vi "数字量输入配置.vi"() -> ()   [LabVIEW 2010] (continued)
              n2465 = local write "单选_第17路"(w82) -> ()
              n2466 = local write "单选_第18路"(w82) -> ()
              n2467 = local write "单选_第19路"(w82) -> ()
              n2468 = local write "单选_第20路"(w82) -> ()
              n2469 = local write "单选_第21路"(w82) -> ()
              n2470 = local write "单选_第22路"(w82) -> ()
              n2471 = local write "单选_第23路"(w82) -> ()
              n2472 = local write "单选_第24路"(w82) -> ()
              n2473 = local write "单选_第25路"(w82) -> ()
              n2474 = local write "单选_第26路"(w83) -> ()
              n2475 = local write "单选_第27路"(w83) -> ()
              n2476 = local write "单选_第28路"(w83) -> ()
              n2477 = local write "单选_第29路"(w83) -> ()
              n2478 = local write "单选_第30路"(w83) -> ()
              n2479 = local write "单选_第31路"(w83) -> ()
              n2480 = local write "单选_第32路"(w83) -> ()
              n2481 = local write "单选_第33路"(w83) -> ()
              n2482 = local write "单选_第34路"(w83) -> ()
              n2483 = local write "单选_第35路"(w83) -> ()
              n2484 = local write "单选_第36路"(w83) -> ()
              n2485 = local write "单选_第37路"(w83) -> ()
              n2486 = local write "单选_第38路"(w83) -> ()
              n2487 = local write "单选_第39路"(w83) -> ()
              n2488 = local write "单选_第40路"(w83) -> ()
              n2489 = local write "单选_第41路"(w83) -> ()
              n2490 = local write "单选_第42路"(w83) -> ()
              n2491 = local write "单选_第43路"(w83) -> ()
              n2492 = local write "单选_第44路"(w83) -> ()
              n2493 = local write "单选_第45路"(w83) -> ()
              n2494 = local write "单选_第46路"(w83) -> ()
              n2495 = local write "单选_第47路"(w83) -> ()
              n2496 = local write "单选_第48路"(w83) -> ()
              n2497 = local write "单选_第49路"(w83) -> ()
              n2498 = local write "单选_第50路"(w83) -> ()
              n2499 = local write "单选_第51路"(w83) -> ()
              n2500 = local write "单选_第52路"(w83) -> ()
              n2501 = local write "单选_第53路"(w83) -> ()
              n2502 = local write "单选_第54路"(w83) -> ()
              n2503 = local write "单选_第55路"(w83) -> ()
              n2504 = local write "单选_第56路"(w83) -> ()
              n2505 = local write "单选_第57路"(w83) -> ()
              n2506 = local write "单选_第58路"(w83) -> ()
              n2507 = local write "单选_第59路"(w83) -> ()
              n2508 = local write "单选_第60路"(w83) -> ()
              n2509 = local write "单选_第61路"(w83) -> ()
              n2510 = local write "单选_第62路"(w83) -> ()
              n2511 = local write "单选_第63路"(w83) -> ()
              n2512 = local write "单选_第64路"(w83) -> ()
              n2513 = local write "单选_第71路"(w83) -> ()
              n2514 = local write "单选_第79路"(w83) -> ()
              n2515 = local write "单选_第65路"(w83) -> ()
              n2516 = local write "单选_第66路"(w83) -> ()
              n2517 = local write "单选_第67路"(w83) -> ()
              n2518 = local write "单选_第68路"(w83) -> ()
              n2519 = local write "单选_第69路"(w83) -> ()
              n2520 = local write "单选_第70路"(w83) -> ()
              n2521 = local write "单选_第72路"(w83) -> ()
              n2522 = local write "单选_第73路"(w83) -> ()
              n2523 = local write "单选_第74路"(w83) -> ()
              n2524 = local write "单选_第75路"(w83) -> ()
              n2525 = local write "单选_第76路"(w83) -> ()
              n2526 = local write "单选_第77路"(w83) -> ()
              n2527 = local write "单选_第78路"(w83) -> ()
              n2528 = local write "单选_第80路"(w83) -> ()
            }
            frame 26 {
              w84 = TRUE
              w85 = FALSE ("单选_第41路")
              n2529 = local write "单选_第1路"(w84) -> ()
              n2530 = local write "单选_第2路"(w84) -> ()
              n2531 = local write "单选_第3路"(w84) -> ()
              n2532 = local write "单选_第4路"(w84) -> ()
              n2533 = local write "单选_第5路"(w84) -> ()
              n2534 = local write "单选_第6路"(w84) -> ()
              n2535 = local write "单选_第7路"(w84) -> ()
              n2536 = local write "单选_第8路"(w84) -> ()
              n2537 = local write "单选_第9路"(w84) -> ()
              n2538 = local write "单选_第10路"(w84) -> ()
              n2539 = local write "单选_第11路"(w84) -> ()
              n2540 = local write "单选_第12路"(w84) -> ()
              n2541 = local write "单选_第13路"(w84) -> ()
              n2542 = local write "单选_第14路"(w84) -> ()
              n2543 = local write "单选_第15路"(w84) -> ()
              n2544 = local write "单选_第16路"(w84) -> ()
              n2545 = local write "单选_第17路"(w84) -> ()
              n2546 = local write "单选_第18路"(w84) -> ()
              n2547 = local write "单选_第19路"(w84) -> ()
              n2548 = local write "单选_第20路"(w84) -> ()
              n2549 = local write "单选_第21路"(w84) -> ()
              n2550 = local write "单选_第22路"(w84) -> ()
              n2551 = local write "单选_第23路"(w84) -> ()
              n2552 = local write "单选_第24路"(w84) -> ()
              n2553 = local write "单选_第25路"(w84) -> ()
              n2554 = local write "单选_第26路"(w84) -> ()
              n2555 = local write "单选_第27路"(w85) -> ()
              n2556 = local write "单选_第28路"(w85) -> ()
              n2557 = local write "单选_第29路"(w85) -> ()
              n2558 = local write "单选_第30路"(w85) -> ()
              n2559 = local write "单选_第31路"(w85) -> ()
              n2560 = local write "单选_第32路"(w85) -> ()
              n2561 = local write "单选_第33路"(w85) -> ()
              n2562 = local write "单选_第34路"(w85) -> ()
              n2563 = local write "单选_第35路"(w85) -> ()
              n2564 = local write "单选_第36路"(w85) -> ()
              n2565 = local write "单选_第37路"(w85) -> ()
              n2566 = local write "单选_第38路"(w85) -> ()
              n2567 = local write "单选_第39路"(w85) -> ()
              n2568 = local write "单选_第40路"(w85) -> ()
              n2569 = local write "单选_第41路"(w85) -> ()
              n2570 = local write "单选_第42路"(w85) -> ()
              n2571 = local write "单选_第43路"(w85) -> ()
              n2572 = local write "单选_第44路"(w85) -> ()
              n2573 = local write "单选_第45路"(w85) -> ()
              n2574 = local write "单选_第46路"(w85) -> ()
              n2575 = local write "单选_第47路"(w85) -> ()
              n2576 = local write "单选_第48路"(w85) -> ()
              n2577 = local write "单选_第49路"(w85) -> ()
              n2578 = local write "单选_第50路"(w85) -> ()
              n2579 = local write "单选_第51路"(w85) -> ()
              n2580 = local write "单选_第52路"(w85) -> ()
              n2581 = local write "单选_第53路"(w85) -> ()
              n2582 = local write "单选_第54路"(w85) -> ()
              n2583 = local write "单选_第55路"(w85) -> ()
              n2584 = local write "单选_第56路"(w85) -> ()
              n2585 = local write "单选_第57路"(w85) -> ()
              n2586 = local write "单选_第58路"(w85) -> ()
              n2587 = local write "单选_第59路"(w85) -> ()
              n2588 = local write "单选_第60路"(w85) -> ()
              n2589 = local write "单选_第61路"(w85) -> ()
              n2590 = local write "单选_第62路"(w85) -> ()
              n2591 = local write "单选_第63路"(w85) -> ()
              n2592 = local write "单选_第64路"(w85) -> ()
              n2593 = local write "单选_第71路"(w85) -> ()
              n2594 = local write "单选_第79路"(w85) -> ()
              n2595 = local write "单选_第65路"(w85) -> ()
              n2596 = local write "单选_第66路"(w85) -> ()
              n2597 = local write "单选_第67路"(w85) -> ()
              n2598 = local write "单选_第68路"(w85) -> ()
              n2599 = local write "单选_第69路"(w85) -> ()
              n2600 = local write "单选_第70路"(w85) -> ()
              n2601 = local write "单选_第72路"(w85) -> ()
              n2602 = local write "单选_第73路"(w85) -> ()
              n2603 = local write "单选_第74路"(w85) -> ()
              n2604 = local write "单选_第75路"(w85) -> ()
              n2605 = local write "单选_第76路"(w85) -> ()
              n2606 = local write "单选_第77路"(w85) -> ()
              n2607 = local write "单选_第78路"(w85) -> ()
              n2608 = local write "单选_第80路"(w85) -> ()
            }
            frame 27 {
              w86 = TRUE
              w87 = FALSE ("单选_第41路")
              n2609 = local write "单选_第1路"(w86) -> ()
              n2610 = local write "单选_第2路"(w86) -> ()
              n2611 = local write "单选_第3路"(w86) -> ()
              n2612 = local write "单选_第4路"(w86) -> ()
              n2613 = local write "单选_第5路"(w86) -> ()
              n2614 = local write "单选_第6路"(w86) -> ()
              n2615 = local write "单选_第7路"(w86) -> ()
              n2616 = local write "单选_第8路"(w86) -> ()
              n2617 = local write "单选_第9路"(w86) -> ()
              n2618 = local write "单选_第10路"(w86) -> ()
              n2619 = local write "单选_第11路"(w86) -> ()
              n2620 = local write "单选_第12路"(w86) -> ()
              n2621 = local write "单选_第13路"(w86) -> ()
              n2622 = local write "单选_第14路"(w86) -> ()
              n2623 = local write "单选_第15路"(w86) -> ()
              n2624 = local write "单选_第16路"(w86) -> ()
              n2625 = local write "单选_第17路"(w86) -> ()
              n2626 = local write "单选_第18路"(w86) -> ()
              n2627 = local write "单选_第19路"(w86) -> ()
              n2628 = local write "单选_第20路"(w86) -> ()
              n2629 = local write "单选_第21路"(w86) -> ()
              n2630 = local write "单选_第22路"(w86) -> ()
              n2631 = local write "单选_第23路"(w86) -> ()
              n2632 = local write "单选_第24路"(w86) -> ()
              n2633 = local write "单选_第25路"(w86) -> ()
              n2634 = local write "单选_第26路"(w86) -> ()
              n2635 = local write "单选_第27路"(w86) -> ()
              n2636 = local write "单选_第28路"(w87) -> ()
              n2637 = local write "单选_第29路"(w87) -> ()
              n2638 = local write "单选_第30路"(w87) -> ()
              n2639 = local write "单选_第31路"(w87) -> ()
              n2640 = local write "单选_第32路"(w87) -> ()
              n2641 = local write "单选_第33路"(w87) -> ()
              n2642 = local write "单选_第34路"(w87) -> ()
              n2643 = local write "单选_第35路"(w87) -> ()
              n2644 = local write "单选_第36路"(w87) -> ()
              n2645 = local write "单选_第37路"(w87) -> ()
              n2646 = local write "单选_第38路"(w87) -> ()
              n2647 = local write "单选_第39路"(w87) -> ()
              n2648 = local write "单选_第40路"(w87) -> ()
              n2649 = local write "单选_第41路"(w87) -> ()
              n2650 = local write "单选_第42路"(w87) -> ()
              n2651 = local write "单选_第43路"(w87) -> ()
              n2652 = local write "单选_第44路"(w87) -> ()
              n2653 = local write "单选_第45路"(w87) -> ()
              n2654 = local write "单选_第46路"(w87) -> ()
              n2655 = local write "单选_第47路"(w87) -> ()
              n2656 = local write "单选_第48路"(w87) -> ()
              n2657 = local write "单选_第49路"(w87) -> ()
              n2658 = local write "单选_第50路"(w87) -> ()
              n2659 = local write "单选_第51路"(w87) -> ()
              n2660 = local write "单选_第52路"(w87) -> ()
              n2661 = local write "单选_第53路"(w87) -> ()
              n2662 = local write "单选_第54路"(w87) -> ()
              n2663 = local write "单选_第55路"(w87) -> ()
              n2664 = local write "单选_第56路"(w87) -> ()
              n2665 = local write "单选_第57路"(w87) -> ()
              n2666 = local write "单选_第58路"(w87) -> ()
              n2667 = local write "单选_第59路"(w87) -> ()
              n2668 = local write "单选_第60路"(w87) -> ()
              n2669 = local write "单选_第61路"(w87) -> ()
              n2670 = local write "单选_第62路"(w87) -> ()
              n2671 = local write "单选_第63路"(w87) -> ()
              n2672 = local write "单选_第64路"(w87) -> ()
              n2673 = local write "单选_第71路"(w87) -> ()
              n2674 = local write "单选_第79路"(w87) -> ()
              n2675 = local write "单选_第65路"(w87) -> ()
              n2676 = local write "单选_第66路"(w87) -> ()
              n2677 = local write "单选_第67路"(w87) -> ()
              n2678 = local write "单选_第68路"(w87) -> ()
              n2679 = local write "单选_第69路"(w87) -> ()
              n2680 = local write "单选_第70路"(w87) -> ()
              n2681 = local write "单选_第72路"(w87) -> ()
              n2682 = local write "单选_第73路"(w87) -> ()
              n2683 = local write "单选_第74路"(w87) -> ()
              n2684 = local write "单选_第75路"(w87) -> ()
              n2685 = local write "单选_第76路"(w87) -> ()
              n2686 = local write "单选_第77路"(w87) -> ()
              n2687 = local write "单选_第78路"(w87) -> ()
              n2688 = local write "单选_第80路"(w87) -> ()
            }
            frame 28 {
              w88 = TRUE
              w89 = FALSE ("单选_第41路")
              n2689 = local write "单选_第1路"(w88) -> ()
              n2690 = local write "单选_第2路"(w88) -> ()
              n2691 = local write "单选_第3路"(w88) -> ()
              n2692 = local write "单选_第4路"(w88) -> ()
              n2693 = local write "单选_第5路"(w88) -> ()
              n2694 = local write "单选_第6路"(w88) -> ()
              n2695 = local write "单选_第7路"(w88) -> ()
              n2696 = local write "单选_第8路"(w88) -> ()
              n2697 = local write "单选_第9路"(w88) -> ()
              n2698 = local write "单选_第10路"(w88) -> ()
              n2699 = local write "单选_第11路"(w88) -> ()
              n2700 = local write "单选_第12路"(w88) -> ()
              n2701 = local write "单选_第13路"(w88) -> ()
              n2702 = local write "单选_第14路"(w88) -> ()
              n2703 = local write "单选_第15路"(w88) -> ()
              n2704 = local write "单选_第16路"(w88) -> ()
              n2705 = local write "单选_第17路"(w88) -> ()
              n2706 = local write "单选_第18路"(w88) -> ()
              n2707 = local write "单选_第19路"(w88) -> ()
              n2708 = local write "单选_第20路"(w88) -> ()
              n2709 = local write "单选_第21路"(w88) -> ()
              n2710 = local write "单选_第22路"(w88) -> ()
              n2711 = local write "单选_第23路"(w88) -> ()
              n2712 = local write "单选_第24路"(w88) -> ()
              n2713 = local write "单选_第25路"(w88) -> ()
              n2714 = local write "单选_第26路"(w88) -> ()
              n2715 = local write "单选_第27路"(w88) -> ()
              n2716 = local write "单选_第28路"(w88) -> ()
              n2717 = local write "单选_第29路"(w89) -> ()
              n2718 = local write "单选_第30路"(w89) -> ()
              n2719 = local write "单选_第31路"(w89) -> ()
              n2720 = local write "单选_第32路"(w89) -> ()
              n2721 = local write "单选_第33路"(w89) -> ()
              n2722 = local write "单选_第34路"(w89) -> ()
              n2723 = local write "单选_第35路"(w89) -> ()
              n2724 = local write "单选_第36路"(w89) -> ()
              n2725 = local write "单选_第37路"(w89) -> ()
              n2726 = local write "单选_第38路"(w89) -> ()
              n2727 = local write "单选_第39路"(w89) -> ()
              n2728 = local write "单选_第40路"(w89) -> ()
              n2729 = local write "单选_第41路"(w89) -> ()
              n2730 = local write "单选_第42路"(w89) -> ()
              n2731 = local write "单选_第43路"(w89) -> ()
              n2732 = local write "单选_第44路"(w89) -> ()
              n2733 = local write "单选_第45路"(w89) -> ()
              n2734 = local write "单选_第46路"(w89) -> ()
              n2735 = local write "单选_第47路"(w89) -> ()
              n2736 = local write "单选_第48路"(w89) -> ()
              n2737 = local write "单选_第49路"(w89) -> ()
              n2738 = local write "单选_第50路"(w89) -> ()
              n2739 = local write "单选_第51路"(w89) -> ()
              n2740 = local write "单选_第52路"(w89) -> ()
              n2741 = local write "单选_第53路"(w89) -> ()
              n2742 = local write "单选_第54路"(w89) -> ()
              n2743 = local write "单选_第55路"(w89) -> ()
              n2744 = local write "单选_第56路"(w89) -> ()
              n2745 = local write "单选_第57路"(w89) -> ()
              n2746 = local write "单选_第58路"(w89) -> ()
              n2747 = local write "单选_第59路"(w89) -> ()
              n2748 = local write "单选_第60路"(w89) -> ()
              n2749 = local write "单选_第61路"(w89) -> ()
              n2750 = local write "单选_第62路"(w89) -> ()
              n2751 = local write "单选_第63路"(w89) -> ()
              n2752 = local write "单选_第64路"(w89) -> ()
              n2753 = local write "单选_第71路"(w89) -> ()
              n2754 = local write "单选_第79路"(w89) -> ()
              n2755 = local write "单选_第65路"(w89) -> ()
              n2756 = local write "单选_第66路"(w89) -> ()
              n2757 = local write "单选_第67路"(w89) -> ()
              n2758 = local write "单选_第68路"(w89) -> ()
              n2759 = local write "单选_第69路"(w89) -> ()
              n2760 = local write "单选_第70路"(w89) -> ()
              n2761 = local write "单选_第72路"(w89) -> ()
              n2762 = local write "单选_第73路"(w89) -> ()
              n2763 = local write "单选_第74路"(w89) -> ()
              n2764 = local write "单选_第75路"(w89) -> ()
              n2765 = local write "单选_第76路"(w89) -> ()
              n2766 = local write "单选_第77路"(w89) -> ()
              n2767 = local write "单选_第78路"(w89) -> ()
              n2768 = local write "单选_第80路"(w89) -> ()
            }
            frame 29 {
              w90 = TRUE
              w91 = FALSE ("单选_第41路")
              n2769 = local write "单选_第1路"(w90) -> ()
              n2770 = local write "单选_第2路"(w90) -> ()
              n2771 = local write "单选_第3路"(w90) -> ()
              n2772 = local write "单选_第4路"(w90) -> ()
              n2773 = local write "单选_第5路"(w90) -> ()
              n2774 = local write "单选_第6路"(w90) -> ()
              n2775 = local write "单选_第7路"(w90) -> ()
              n2776 = local write "单选_第8路"(w90) -> ()
              n2777 = local write "单选_第9路"(w90) -> ()
              n2778 = local write "单选_第10路"(w90) -> ()
              n2779 = local write "单选_第11路"(w90) -> ()
              n2780 = local write "单选_第12路"(w90) -> ()
              n2781 = local write "单选_第13路"(w90) -> ()
              n2782 = local write "单选_第14路"(w90) -> ()
              n2783 = local write "单选_第15路"(w90) -> ()
              n2784 = local write "单选_第16路"(w90) -> ()
              n2785 = local write "单选_第17路"(w90) -> ()
              n2786 = local write "单选_第18路"(w90) -> ()
              n2787 = local write "单选_第19路"(w90) -> ()
              n2788 = local write "单选_第20路"(w90) -> ()
              n2789 = local write "单选_第21路"(w90) -> ()
              n2790 = local write "单选_第22路"(w90) -> ()
              n2791 = local write "单选_第23路"(w90) -> ()
              n2792 = local write "单选_第24路"(w90) -> ()
              n2793 = local write "单选_第25路"(w90) -> ()
              n2794 = local write "单选_第26路"(w90) -> ()
              n2795 = local write "单选_第27路"(w90) -> ()
              n2796 = local write "单选_第28路"(w90) -> ()
              n2797 = local write "单选_第29路"(w90) -> ()
              n2798 = local write "单选_第30路"(w91) -> ()
              n2799 = local write "单选_第31路"(w91) -> ()
              n2800 = local write "单选_第32路"(w91) -> ()
              n2801 = local write "单选_第33路"(w91) -> ()
              n2802 = local write "单选_第34路"(w91) -> ()
              n2803 = local write "单选_第35路"(w91) -> ()
              n2804 = local write "单选_第36路"(w91) -> ()
              n2805 = local write "单选_第37路"(w91) -> ()
              n2806 = local write "单选_第38路"(w91) -> ()
              n2807 = local write "单选_第39路"(w91) -> ()
              n2808 = local write "单选_第40路"(w91) -> ()
              n2809 = local write "单选_第41路"(w91) -> ()
              n2810 = local write "单选_第42路"(w91) -> ()
              n2811 = local write "单选_第43路"(w91) -> ()
              n2812 = local write "单选_第44路"(w91) -> ()
              n2813 = local write "单选_第45路"(w91) -> ()
              n2814 = local write "单选_第46路"(w91) -> ()
              n2815 = local write "单选_第47路"(w91) -> ()
              n2816 = local write "单选_第48路"(w91) -> ()
              n2817 = local write "单选_第49路"(w91) -> ()
              n2818 = local write "单选_第50路"(w91) -> ()
              n2819 = local write "单选_第51路"(w91) -> ()
              n2820 = local write "单选_第52路"(w91) -> ()
              n2821 = local write "单选_第53路"(w91) -> ()
              n2822 = local write "单选_第54路"(w91) -> ()
              n2823 = local write "单选_第55路"(w91) -> ()
              n2824 = local write "单选_第56路"(w91) -> ()
              n2825 = local write "单选_第57路"(w91) -> ()
              n2826 = local write "单选_第58路"(w91) -> ()
              n2827 = local write "单选_第59路"(w91) -> ()
              n2828 = local write "单选_第60路"(w91) -> ()
              n2829 = local write "单选_第61路"(w91) -> ()
              n2830 = local write "单选_第62路"(w91) -> ()
              n2831 = local write "单选_第63路"(w91) -> ()
              n2832 = local write "单选_第64路"(w91) -> ()
              n2833 = local write "单选_第71路"(w91) -> ()
              n2834 = local write "单选_第79路"(w91) -> ()
              n2835 = local write "单选_第65路"(w91) -> ()
              n2836 = local write "单选_第66路"(w91) -> ()
              n2837 = local write "单选_第67路"(w91) -> ()
              n2838 = local write "单选_第68路"(w91) -> ()
              n2839 = local write "单选_第69路"(w91) -> ()
              n2840 = local write "单选_第70路"(w91) -> ()
              n2841 = local write "单选_第72路"(w91) -> ()
              n2842 = local write "单选_第73路"(w91) -> ()
              n2843 = local write "单选_第74路"(w91) -> ()
              n2844 = local write "单选_第75路"(w91) -> ()
              n2845 = local write "单选_第76路"(w91) -> ()
              n2846 = local write "单选_第77路"(w91) -> ()
              n2847 = local write "单选_第78路"(w91) -> ()
              n2848 = local write "单选_第80路"(w91) -> ()
            }
            frame 30 {
              w92 = TRUE
              w93 = FALSE ("单选_第41路")
              n2849 = local write "单选_第1路"(w92) -> ()
              n2850 = local write "单选_第2路"(w92) -> ()
              n2851 = local write "单选_第3路"(w92) -> ()
              n2852 = local write "单选_第4路"(w92) -> ()
              n2853 = local write "单选_第5路"(w92) -> ()
              n2854 = local write "单选_第6路"(w92) -> ()
              n2855 = local write "单选_第7路"(w92) -> ()
              n2856 = local write "单选_第8路"(w92) -> ()
              n2857 = local write "单选_第9路"(w92) -> ()
              n2858 = local write "单选_第10路"(w92) -> ()
              n2859 = local write "单选_第11路"(w92) -> ()
              n2860 = local write "单选_第12路"(w92) -> ()
              n2861 = local write "单选_第13路"(w92) -> ()
              n2862 = local write "单选_第14路"(w92) -> ()
              n2863 = local write "单选_第15路"(w92) -> ()
              n2864 = local write "单选_第16路"(w92) -> ()
              n2865 = local write "单选_第17路"(w92) -> ()
              n2866 = local write "单选_第18路"(w92) -> ()
              n2867 = local write "单选_第19路"(w92) -> ()
              n2868 = local write "单选_第20路"(w92) -> ()
              n2869 = local write "单选_第21路"(w92) -> ()
              n2870 = local write "单选_第22路"(w92) -> ()
              n2871 = local write "单选_第23路"(w92) -> ()
              n2872 = local write "单选_第24路"(w92) -> ()
              n2873 = local write "单选_第25路"(w92) -> ()
              n2874 = local write "单选_第26路"(w92) -> ()
              n2875 = local write "单选_第27路"(w92) -> ()
              n2876 = local write "单选_第28路"(w92) -> ()
              n2877 = local write "单选_第29路"(w92) -> ()
              n2878 = local write "单选_第30路"(w92) -> ()
              n2879 = local write "单选_第31路"(w93) -> ()
              n2880 = local write "单选_第32路"(w93) -> ()
              n2881 = local write "单选_第33路"(w93) -> ()
              n2882 = local write "单选_第34路"(w93) -> ()
              n2883 = local write "单选_第35路"(w93) -> ()
              n2884 = local write "单选_第36路"(w93) -> ()
              n2885 = local write "单选_第37路"(w93) -> ()
              n2886 = local write "单选_第38路"(w93) -> ()
              n2887 = local write "单选_第39路"(w93) -> ()
              n2888 = local write "单选_第40路"(w93) -> ()
              n2889 = local write "单选_第41路"(w93) -> ()
              n2890 = local write "单选_第42路"(w93) -> ()
              n2891 = local write "单选_第43路"(w93) -> ()
              n2892 = local write "单选_第44路"(w93) -> ()
              n2893 = local write "单选_第45路"(w93) -> ()
              n2894 = local write "单选_第46路"(w93) -> ()
              n2895 = local write "单选_第47路"(w93) -> ()
              n2896 = local write "单选_第48路"(w93) -> ()
              n2897 = local write "单选_第49路"(w93) -> ()
              n2898 = local write "单选_第50路"(w93) -> ()
              n2899 = local write "单选_第51路"(w93) -> ()
              n2900 = local write "单选_第52路"(w93) -> ()
              n2901 = local write "单选_第53路"(w93) -> ()
              n2902 = local write "单选_第54路"(w93) -> ()
              n2903 = local write "单选_第55路"(w93) -> ()
              n2904 = local write "单选_第56路"(w93) -> ()
              n2905 = local write "单选_第57路"(w93) -> ()
              n2906 = local write "单选_第58路"(w93) -> ()
              n2907 = local write "单选_第59路"(w93) -> ()
              n2908 = local write "单选_第60路"(w93) -> ()
              n2909 = local write "单选_第61路"(w93) -> ()
              n2910 = local write "单选_第62路"(w93) -> ()
              n2911 = local write "单选_第63路"(w93) -> ()
              n2912 = local write "单选_第64路"(w93) -> ()
              n2913 = local write "单选_第71路"(w93) -> ()
              n2914 = local write "单选_第79路"(w93) -> ()
              n2915 = local write "单选_第65路"(w93) -> ()
              n2916 = local write "单选_第66路"(w93) -> ()
              n2917 = local write "单选_第67路"(w93) -> ()
              n2918 = local write "单选_第68路"(w93) -> ()
              n2919 = local write "单选_第69路"(w93) -> ()
              n2920 = local write "单选_第70路"(w93) -> ()
              n2921 = local write "单选_第72路"(w93) -> ()
              n2922 = local write "单选_第73路"(w93) -> ()
              n2923 = local write "单选_第74路"(w93) -> ()
              n2924 = local write "单选_第75路"(w93) -> ()
              n2925 = local write "单选_第76路"(w93) -> ()
              n2926 = local write "单选_第77路"(w93) -> ()
              n2927 = local write "单选_第78路"(w93) -> ()
              n2928 = local write "单选_第80路"(w93) -> ()
            }
            frame 31 {
              w94 = TRUE
              w95 = FALSE ("单选_第41路")
              n2929 = local write "单选_第1路"(w94) -> ()
              n2930 = local write "单选_第2路"(w94) -> ()
              n2931 = local write "单选_第3路"(w94) -> ()
              n2932 = local write "单选_第4路"(w94) -> ()
              n2933 = local write "单选_第5路"(w94) -> ()
              n2934 = local write "单选_第6路"(w94) -> ()
              n2935 = local write "单选_第7路"(w94) -> ()
              n2936 = local write "单选_第8路"(w94) -> ()
              n2937 = local write "单选_第9路"(w94) -> ()
              n2938 = local write "单选_第10路"(w94) -> ()
              n2939 = local write "单选_第11路"(w94) -> ()
              n2940 = local write "单选_第12路"(w94) -> ()
              n2941 = local write "单选_第13路"(w94) -> ()
              n2942 = local write "单选_第14路"(w94) -> ()
              n2943 = local write "单选_第15路"(w94) -> ()
              n2944 = local write "单选_第16路"(w94) -> ()
              n2945 = local write "单选_第17路"(w94) -> ()
              n2946 = local write "单选_第18路"(w94) -> ()
              n2947 = local write "单选_第19路"(w94) -> ()
              n2948 = local write "单选_第20路"(w94) -> ()
              n2949 = local write "单选_第21路"(w94) -> ()
              n2950 = local write "单选_第22路"(w94) -> ()
              n2951 = local write "单选_第23路"(w94) -> ()
              n2952 = local write "单选_第24路"(w94) -> ()
              n2953 = local write "单选_第25路"(w94) -> ()
              n2954 = local write "单选_第26路"(w94) -> ()
              n2955 = local write "单选_第27路"(w94) -> ()
              n2956 = local write "单选_第28路"(w94) -> ()
              n2957 = local write "单选_第29路"(w94) -> ()
              n2958 = local write "单选_第30路"(w94) -> ()
              n2959 = local write "单选_第31路"(w94) -> ()
              n2960 = local write "单选_第32路"(w95) -> ()
              n2961 = local write "单选_第33路"(w95) -> ()
              n2962 = local write "单选_第34路"(w95) -> ()
              n2963 = local write "单选_第35路"(w95) -> ()
              n2964 = local write "单选_第36路"(w95) -> ()
              n2965 = local write "单选_第37路"(w95) -> ()
              n2966 = local write "单选_第38路"(w95) -> ()
              n2967 = local write "单选_第39路"(w95) -> ()
              n2968 = local write "单选_第40路"(w95) -> ()
              n2969 = local write "单选_第41路"(w95) -> ()
              n2970 = local write "单选_第42路"(w95) -> ()
              n2971 = local write "单选_第43路"(w95) -> ()
              n2972 = local write "单选_第44路"(w95) -> ()
              n2973 = local write "单选_第45路"(w95) -> ()
              n2974 = local write "单选_第46路"(w95) -> ()
              n2975 = local write "单选_第47路"(w95) -> ()
              n2976 = local write "单选_第48路"(w95) -> ()
              n2977 = local write "单选_第49路"(w95) -> ()
              n2978 = local write "单选_第50路"(w95) -> ()
              n2979 = local write "单选_第51路"(w95) -> ()
              n2980 = local write "单选_第52路"(w95) -> ()
              n2981 = local write "单选_第53路"(w95) -> ()
              n2982 = local write "单选_第54路"(w95) -> ()
              n2983 = local write "单选_第55路"(w95) -> ()
              n2984 = local write "单选_第56路"(w95) -> ()
              n2985 = local write "单选_第57路"(w95) -> ()
              n2986 = local write "单选_第58路"(w95) -> ()
              n2987 = local write "单选_第59路"(w95) -> ()
              n2988 = local write "单选_第60路"(w95) -> ()
              n2989 = local write "单选_第61路"(w95) -> ()
              n2990 = local write "单选_第62路"(w95) -> ()
              n2991 = local write "单选_第63路"(w95) -> ()
              n2992 = local write "单选_第64路"(w95) -> ()
              n2993 = local write "单选_第71路"(w95) -> ()
              n2994 = local write "单选_第79路"(w95) -> ()
              n2995 = local write "单选_第65路"(w95) -> ()
              n2996 = local write "单选_第66路"(w95) -> ()
              n2997 = local write "单选_第67路"(w95) -> ()
              n2998 = local write "单选_第68路"(w95) -> ()
              n2999 = local write "单选_第69路"(w95) -> ()
              n3000 = local write "单选_第70路"(w95) -> ()
              n3001 = local write "单选_第72路"(w95) -> ()
              n3002 = local write "单选_第73路"(w95) -> ()
              n3003 = local write "单选_第74路"(w95) -> ()
              n3004 = local write "单选_第75路"(w95) -> ()
              n3005 = local write "单选_第76路"(w95) -> ()
              n3006 = local write "单选_第77路"(w95) -> ()
              n3007 = local write "单选_第78路"(w95) -> ()
              n3008 = local write "单选_第80路"(w95) -> ()
            }
            frame 32 {
              w96 = TRUE
              w97 = FALSE ("单选_第41路")
              n3009 = local write "单选_第1路"(w96) -> ()
              n3010 = local write "单选_第2路"(w96) -> ()
              n3011 = local write "单选_第3路"(w96) -> ()
              n3012 = local write "单选_第4路"(w96) -> ()
              n3013 = local write "单选_第5路"(w96) -> ()
              n3014 = local write "单选_第6路"(w96) -> ()
              n3015 = local write "单选_第7路"(w96) -> ()
              n3016 = local write "单选_第8路"(w96) -> ()
              n3017 = local write "单选_第9路"(w96) -> ()
              n3018 = local write "单选_第10路"(w96) -> ()
              n3019 = local write "单选_第11路"(w96) -> ()
              n3020 = local write "单选_第12路"(w96) -> ()
              n3021 = local write "单选_第13路"(w96) -> ()
              n3022 = local write "单选_第14路"(w96) -> ()
              n3023 = local write "单选_第15路"(w96) -> ()
              n3024 = local write "单选_第16路"(w96) -> ()
              n3025 = local write "单选_第17路"(w96) -> ()
              n3026 = local write "单选_第18路"(w96) -> ()
              n3027 = local write "单选_第19路"(w96) -> ()
              n3028 = local write "单选_第20路"(w96) -> ()
              n3029 = local write "单选_第21路"(w96) -> ()
              n3030 = local write "单选_第22路"(w96) -> ()
              n3031 = local write "单选_第23路"(w96) -> ()
              n3032 = local write "单选_第24路"(w96) -> ()
              n3033 = local write "单选_第25路"(w96) -> ()
              n3034 = local write "单选_第26路"(w96) -> ()
              n3035 = local write "单选_第27路"(w96) -> ()
              n3036 = local write "单选_第28路"(w96) -> ()
              n3037 = local write "单选_第29路"(w96) -> ()
              n3038 = local write "单选_第30路"(w96) -> ()
              n3039 = local write "单选_第31路"(w96) -> ()
              n3040 = local write "单选_第32路"(w96) -> ()
              n3041 = local write "单选_第33路"(w97) -> ()
              n3042 = local write "单选_第34路"(w97) -> ()
              n3043 = local write "单选_第35路"(w97) -> ()
              n3044 = local write "单选_第36路"(w97) -> ()
              n3045 = local write "单选_第37路"(w97) -> ()
              n3046 = local write "单选_第38路"(w97) -> ()
              n3047 = local write "单选_第39路"(w97) -> ()
              n3048 = local write "单选_第40路"(w97) -> ()
              n3049 = local write "单选_第41路"(w97) -> ()
              n3050 = local write "单选_第42路"(w97) -> ()
              n3051 = local write "单选_第43路"(w97) -> ()
              n3052 = local write "单选_第44路"(w97) -> ()
              n3053 = local write "单选_第45路"(w97) -> ()
              n3054 = local write "单选_第46路"(w97) -> ()
              n3055 = local write "单选_第47路"(w97) -> ()
              n3056 = local write "单选_第48路"(w97) -> ()
              n3057 = local write "单选_第49路"(w97) -> ()
              n3058 = local write "单选_第50路"(w97) -> ()
              n3059 = local write "单选_第51路"(w97) -> ()
              n3060 = local write "单选_第52路"(w97) -> ()
              n3061 = local write "单选_第53路"(w97) -> ()
              n3062 = local write "单选_第54路"(w97) -> ()
              n3063 = local write "单选_第55路"(w97) -> ()
              n3064 = local write "单选_第56路"(w97) -> ()
              n3065 = local write "单选_第57路"(w97) -> ()
              n3066 = local write "单选_第58路"(w97) -> ()
              n3067 = local write "单选_第59路"(w97) -> ()
              n3068 = local write "单选_第60路"(w97) -> ()
              n3069 = local write "单选_第61路"(w97) -> ()
              n3070 = local write "单选_第62路"(w97) -> ()
              n3071 = local write "单选_第63路"(w97) -> ()
              n3072 = local write "单选_第64路"(w97) -> ()
              n3073 = local write "单选_第71路"(w97) -> ()
              n3074 = local write "单选_第79路"(w97) -> ()
              n3075 = local write "单选_第65路"(w97) -> ()
              n3076 = local write "单选_第66路"(w97) -> ()
              n3077 = local write "单选_第67路"(w97) -> ()
              n3078 = local write "单选_第68路"(w97) -> ()
              n3079 = local write "单选_第69路"(w97) -> ()
              n3080 = local write "单选_第70路"(w97) -> ()
              n3081 = local write "单选_第72路"(w97) -> ()
              n3082 = local write "单选_第73路"(w97) -> ()
              n3083 = local write "单选_第74路"(w97) -> ()
              n3084 = local write "单选_第75路"(w97) -> ()
              n3085 = local write "单选_第76路"(w97) -> ()
              n3086 = local write "单选_第77路"(w97) -> ()
              n3087 = local write "单选_第78路"(w97) -> ()
              n3088 = local write "单选_第80路"(w97) -> ()
            }
            frame 33 {
              w98 = TRUE
              w99 = FALSE ("单选_第41路")
              n3089 = local write "单选_第1路"(w98) -> ()
              n3090 = local write "单选_第2路"(w98) -> ()
              n3091 = local write "单选_第3路"(w98) -> ()
              n3092 = local write "单选_第4路"(w98) -> ()
              n3093 = local write "单选_第5路"(w98) -> ()
              n3094 = local write "单选_第6路"(w98) -> ()
              n3095 = local write "单选_第7路"(w98) -> ()
              n3096 = local write "单选_第8路"(w98) -> ()
              n3097 = local write "单选_第9路"(w98) -> ()
              n3098 = local write "单选_第10路"(w98) -> ()
              n3099 = local write "单选_第11路"(w98) -> ()
              n3100 = local write "单选_第12路"(w98) -> ()
              n3101 = local write "单选_第13路"(w98) -> ()
              n3102 = local write "单选_第14路"(w98) -> ()
              n3103 = local write "单选_第15路"(w98) -> ()
              n3104 = local write "单选_第16路"(w98) -> ()
              n3105 = local write "单选_第17路"(w98) -> ()
              n3106 = local write "单选_第18路"(w98) -> ()
              n3107 = local write "单选_第19路"(w98) -> ()
              n3108 = local write "单选_第20路"(w98) -> ()
              n3109 = local write "单选_第21路"(w98) -> ()
              n3110 = local write "单选_第22路"(w98) -> ()
              n3111 = local write "单选_第23路"(w98) -> ()
              n3112 = local write "单选_第24路"(w98) -> ()
              n3113 = local write "单选_第25路"(w98) -> ()
              n3114 = local write "单选_第26路"(w98) -> ()
              n3115 = local write "单选_第27路"(w98) -> ()
              n3116 = local write "单选_第28路"(w98) -> ()
              n3117 = local write "单选_第29路"(w98) -> ()
              n3118 = local write "单选_第30路"(w98) -> ()
              n3119 = local write "单选_第31路"(w98) -> ()
              n3120 = local write "单选_第32路"(w98) -> ()
              n3121 = local write "单选_第33路"(w98) -> ()
              n3122 = local write "单选_第34路"(w99) -> ()
              n3123 = local write "单选_第35路"(w99) -> ()
              n3124 = local write "单选_第36路"(w99) -> ()
              n3125 = local write "单选_第37路"(w99) -> ()
              n3126 = local write "单选_第38路"(w99) -> ()
              n3127 = local write "单选_第39路"(w99) -> ()
              n3128 = local write "单选_第40路"(w99) -> ()
              n3129 = local write "单选_第41路"(w99) -> ()
              n3130 = local write "单选_第42路"(w99) -> ()
              n3131 = local write "单选_第43路"(w99) -> ()
              n3132 = local write "单选_第44路"(w99) -> ()
              n3133 = local write "单选_第45路"(w99) -> ()
              n3134 = local write "单选_第46路"(w99) -> ()
              n3135 = local write "单选_第47路"(w99) -> ()
              n3136 = local write "单选_第48路"(w99) -> ()
              n3137 = local write "单选_第49路"(w99) -> ()
              n3138 = local write "单选_第50路"(w99) -> ()
              n3139 = local write "单选_第51路"(w99) -> ()
              n3140 = local write "单选_第52路"(w99) -> ()
              n3141 = local write "单选_第53路"(w99) -> ()
              n3142 = local write "单选_第54路"(w99) -> ()
              n3143 = local write "单选_第55路"(w99) -> ()
              n3144 = local write "单选_第56路"(w99) -> ()
              n3145 = local write "单选_第57路"(w99) -> ()
              n3146 = local write "单选_第58路"(w99) -> ()
              n3147 = local write "单选_第59路"(w99) -> ()
              n3148 = local write "单选_第60路"(w99) -> ()
              n3149 = local write "单选_第61路"(w99) -> ()
              n3150 = local write "单选_第62路"(w99) -> ()
              n3151 = local write "单选_第63路"(w99) -> ()
              n3152 = local write "单选_第64路"(w99) -> ()
              n3153 = local write "单选_第71路"(w99) -> ()
              n3154 = local write "单选_第79路"(w99) -> ()
              n3155 = local write "单选_第65路"(w99) -> ()
              n3156 = local write "单选_第66路"(w99) -> ()
              n3157 = local write "单选_第67路"(w99) -> ()
              n3158 = local write "单选_第68路"(w99) -> ()
              n3159 = local write "单选_第69路"(w99) -> ()
              n3160 = local write "单选_第70路"(w99) -> ()
              n3161 = local write "单选_第72路"(w99) -> ()
              n3162 = local write "单选_第73路"(w99) -> ()
              n3163 = local write "单选_第74路"(w99) -> ()
              n3164 = local write "单选_第75路"(w99) -> ()
              n3165 = local write "单选_第76路"(w99) -> ()
              n3166 = local write "单选_第77路"(w99) -> ()
              n3167 = local write "单选_第78路"(w99) -> ()
              n3168 = local write "单选_第80路"(w99) -> ()
            }
            frame 34 {
              w100 = TRUE
              w101 = FALSE ("单选_第41路")
              n3169 = local write "单选_第1路"(w100) -> ()
              n3170 = local write "单选_第2路"(w100) -> ()
              n3171 = local write "单选_第3路"(w100) -> ()
              n3172 = local write "单选_第4路"(w100) -> ()
              n3173 = local write "单选_第5路"(w100) -> ()
              n3174 = local write "单选_第6路"(w100) -> ()
              n3175 = local write "单选_第7路"(w100) -> ()
              n3176 = local write "单选_第8路"(w100) -> ()
              n3177 = local write "单选_第9路"(w100) -> ()
              n3178 = local write "单选_第10路"(w100) -> ()
              n3179 = local write "单选_第11路"(w100) -> ()
              n3180 = local write "单选_第12路"(w100) -> ()
              n3181 = local write "单选_第13路"(w100) -> ()
              n3182 = local write "单选_第14路"(w100) -> ()
              n3183 = local write "单选_第15路"(w100) -> ()
              n3184 = local write "单选_第16路"(w100) -> ()
              n3185 = local write "单选_第17路"(w100) -> ()
              n3186 = local write "单选_第18路"(w100) -> ()
              n3187 = local write "单选_第19路"(w100) -> ()
              n3188 = local write "单选_第20路"(w100) -> ()
              n3189 = local write "单选_第21路"(w100) -> ()
              n3190 = local write "单选_第22路"(w100) -> ()
              n3191 = local write "单选_第23路"(w100) -> ()
              n3192 = local write "单选_第24路"(w100) -> ()
              n3193 = local write "单选_第25路"(w100) -> ()
              n3194 = local write "单选_第26路"(w100) -> ()
              n3195 = local write "单选_第27路"(w100) -> ()
              n3196 = local write "单选_第28路"(w100) -> ()
              n3197 = local write "单选_第29路"(w100) -> ()
              n3198 = local write "单选_第30路"(w100) -> ()
              n3199 = local write "单选_第31路"(w100) -> ()
              n3200 = local write "单选_第32路"(w100) -> ()
              n3201 = local write "单选_第33路"(w100) -> ()
              n3202 = local write "单选_第34路"(w100) -> ()
              n3203 = local write "单选_第35路"(w101) -> ()
              n3204 = local write "单选_第36路"(w101) -> ()
              n3205 = local write "单选_第37路"(w101) -> ()
              n3206 = local write "单选_第38路"(w101) -> ()
              n3207 = local write "单选_第39路"(w101) -> ()
              n3208 = local write "单选_第40路"(w101) -> ()
              n3209 = local write "单选_第41路"(w101) -> ()
              n3210 = local write "单选_第42路"(w101) -> ()
              n3211 = local write "单选_第43路"(w101) -> ()
              n3212 = local write "单选_第44路"(w101) -> ()
              n3213 = local write "单选_第45路"(w101) -> ()
              n3214 = local write "单选_第46路"(w101) -> ()
              n3215 = local write "单选_第47路"(w101) -> ()
              n3216 = local write "单选_第48路"(w101) -> ()
              n3217 = local write "单选_第49路"(w101) -> ()
              n3218 = local write "单选_第50路"(w101) -> ()
              n3219 = local write "单选_第51路"(w101) -> ()
              n3220 = local write "单选_第52路"(w101) -> ()
              n3221 = local write "单选_第53路"(w101) -> ()
              n3222 = local write "单选_第54路"(w101) -> ()
              n3223 = local write "单选_第55路"(w101) -> ()
              n3224 = local write "单选_第56路"(w101) -> ()
              n3225 = local write "单选_第57路"(w101) -> ()
              n3226 = local write "单选_第58路"(w101) -> ()
              n3227 = local write "单选_第59路"(w101) -> ()
              n3228 = local write "单选_第60路"(w101) -> ()
              n3229 = local write "单选_第61路"(w101) -> ()
              n3230 = local write "单选_第62路"(w101) -> ()
              n3231 = local write "单选_第63路"(w101) -> ()
              n3232 = local write "单选_第64路"(w101) -> ()
              n3233 = local write "单选_第71路"(w101) -> ()
              n3234 = local write "单选_第79路"(w101) -> ()
              n3235 = local write "单选_第65路"(w101) -> ()
              n3236 = local write "单选_第66路"(w101) -> ()
              n3237 = local write "单选_第67路"(w101) -> ()
              n3238 = local write "单选_第68路"(w101) -> ()
              n3239 = local write "单选_第69路"(w101) -> ()
              n3240 = local write "单选_第70路"(w101) -> ()
              n3241 = local write "单选_第72路"(w101) -> ()
              n3242 = local write "单选_第73路"(w101) -> ()
              n3243 = local write "单选_第74路"(w101) -> ()
              n3244 = local write "单选_第75路"(w101) -> ()
              n3245 = local write "单选_第76路"(w101) -> ()
              n3246 = local write "单选_第77路"(w101) -> ()
              n3247 = local write "单选_第78路"(w101) -> ()
              n3248 = local write "单选_第80路"(w101) -> ()
            }
            frame 35 {
              w102 = TRUE
              w103 = FALSE ("单选_第41路")
              n3249 = local write "单选_第1路"(w102) -> ()
              n3250 = local write "单选_第2路"(w102) -> ()
              n3251 = local write "单选_第3路"(w102) -> ()
              n3252 = local write "单选_第4路"(w102) -> ()
              n3253 = local write "单选_第5路"(w102) -> ()
              n3254 = local write "单选_第6路"(w102) -> ()
              n3255 = local write "单选_第7路"(w102) -> ()
              n3256 = local write "单选_第8路"(w102) -> ()
              n3257 = local write "单选_第9路"(w102) -> ()
              n3258 = local write "单选_第10路"(w102) -> ()
              n3259 = local write "单选_第11路"(w102) -> ()
              n3260 = local write "单选_第12路"(w102) -> ()
              n3261 = local write "单选_第13路"(w102) -> ()
              n3262 = local write "单选_第14路"(w102) -> ()
              n3263 = local write "单选_第15路"(w102) -> ()
              n3264 = local write "单选_第16路"(w102) -> ()
              n3265 = local write "单选_第17路"(w102) -> ()
              n3266 = local write "单选_第18路"(w102) -> ()
              n3267 = local write "单选_第19路"(w102) -> ()
              n3268 = local write "单选_第20路"(w102) -> ()
              n3269 = local write "单选_第21路"(w102) -> ()
              n3270 = local write "单选_第22路"(w102) -> ()
              n3271 = local write "单选_第23路"(w102) -> ()
              n3272 = local write "单选_第24路"(w102) -> ()
              n3273 = local write "单选_第25路"(w102) -> ()
              n3274 = local write "单选_第26路"(w102) -> ()
              n3275 = local write "单选_第27路"(w102) -> ()
              n3276 = local write "单选_第28路"(w102) -> ()
              n3277 = local write "单选_第29路"(w102) -> ()
              n3278 = local write "单选_第30路"(w102) -> ()
              n3279 = local write "单选_第31路"(w102) -> ()
              n3280 = local write "单选_第32路"(w102) -> ()
              n3281 = local write "单选_第33路"(w102) -> ()
              n3282 = local write "单选_第34路"(w102) -> ()
              n3283 = local write "单选_第35路"(w102) -> ()
              n3284 = local write "单选_第36路"(w103) -> ()
              n3285 = local write "单选_第37路"(w103) -> ()
              n3286 = local write "单选_第38路"(w103) -> ()
              n3287 = local write "单选_第39路"(w103) -> ()
              n3288 = local write "单选_第40路"(w103) -> ()
              n3289 = local write "单选_第41路"(w103) -> ()
              n3290 = local write "单选_第42路"(w103) -> ()
              n3291 = local write "单选_第43路"(w103) -> ()
              n3292 = local write "单选_第44路"(w103) -> ()
              n3293 = local write "单选_第45路"(w103) -> ()
              n3294 = local write "单选_第46路"(w103) -> ()
              n3295 = local write "单选_第47路"(w103) -> ()
              n3296 = local write "单选_第48路"(w103) -> ()
              n3297 = local write "单选_第49路"(w103) -> ()
              n3298 = local write "单选_第50路"(w103) -> ()
              n3299 = local write "单选_第51路"(w103) -> ()
              n3300 = local write "单选_第52路"(w103) -> ()
              n3301 = local write "单选_第53路"(w103) -> ()
              n3302 = local write "单选_第54路"(w103) -> ()
              n3303 = local write "单选_第55路"(w103) -> ()
              n3304 = local write "单选_第56路"(w103) -> ()
              n3305 = local write "单选_第57路"(w103) -> ()
              n3306 = local write "单选_第58路"(w103) -> ()
              n3307 = local write "单选_第59路"(w103) -> ()
              n3308 = local write "单选_第60路"(w103) -> ()
              n3309 = local write "单选_第61路"(w103) -> ()
              n3310 = local write "单选_第62路"(w103) -> ()
              n3311 = local write "单选_第63路"(w103) -> ()
              n3312 = local write "单选_第64路"(w103) -> ()
              n3313 = local write "单选_第71路"(w103) -> ()
              n3314 = local write "单选_第79路"(w103) -> ()
              n3315 = local write "单选_第65路"(w103) -> ()
              n3316 = local write "单选_第66路"(w103) -> ()
              n3317 = local write "单选_第67路"(w103) -> ()
              n3318 = local write "单选_第68路"(w103) -> ()
              n3319 = local write "单选_第69路"(w103) -> ()
              n3320 = local write "单选_第70路"(w103) -> ()
              n3321 = local write "单选_第72路"(w103) -> ()
              n3322 = local write "单选_第73路"(w103) -> ()
              n3323 = local write "单选_第74路"(w103) -> ()
              n3324 = local write "单选_第75路"(w103) -> ()
              n3325 = local write "单选_第76路"(w103) -> ()
              n3326 = local write "单选_第77路"(w103) -> ()
              n3327 = local write "单选_第78路"(w103) -> ()
              n3328 = local write "单选_第80路"(w103) -> ()
            }
            frame 36 {
              w104 = TRUE
              w105 = FALSE ("单选_第41路")
              n3329 = local write "单选_第1路"(w104) -> ()
              n3330 = local write "单选_第2路"(w104) -> ()
              n3331 = local write "单选_第3路"(w104) -> ()
              n3332 = local write "单选_第4路"(w104) -> ()
              n3333 = local write "单选_第5路"(w104) -> ()
              n3334 = local write "单选_第6路"(w104) -> ()
              n3335 = local write "单选_第7路"(w104) -> ()
              n3336 = local write "单选_第8路"(w104) -> ()
              n3337 = local write "单选_第9路"(w104) -> ()
              n3338 = local write "单选_第10路"(w104) -> ()
              n3339 = local write "单选_第11路"(w104) -> ()
              n3340 = local write "单选_第12路"(w104) -> ()
              n3341 = local write "单选_第13路"(w104) -> ()
              n3342 = local write "单选_第14路"(w104) -> ()
              n3343 = local write "单选_第15路"(w104) -> ()
              n3344 = local write "单选_第16路"(w104) -> ()
              n3345 = local write "单选_第17路"(w104) -> ()
              n3346 = local write "单选_第18路"(w104) -> ()
              n3347 = local write "单选_第19路"(w104) -> ()
              n3348 = local write "单选_第20路"(w104) -> ()
              n3349 = local write "单选_第21路"(w104) -> ()
              n3350 = local write "单选_第22路"(w104) -> ()
              n3351 = local write "单选_第23路"(w104) -> ()
              n3352 = local write "单选_第24路"(w104) -> ()
              n3353 = local write "单选_第25路"(w104) -> ()
              n3354 = local write "单选_第26路"(w104) -> ()
              n3355 = local write "单选_第27路"(w104) -> ()
              n3356 = local write "单选_第28路"(w104) -> ()
              n3357 = local write "单选_第29路"(w104) -> ()
              n3358 = local write "单选_第30路"(w104) -> ()
              n3359 = local write "单选_第31路"(w104) -> ()
              n3360 = local write "单选_第32路"(w104) -> ()
              n3361 = local write "单选_第33路"(w104) -> ()
              n3362 = local write "单选_第34路"(w104) -> ()
              n3363 = local write "单选_第35路"(w104) -> ()
              n3364 = local write "单选_第36路"(w104) -> ()
              n3365 = local write "单选_第37路"(w105) -> ()
              n3366 = local write "单选_第38路"(w105) -> ()
              n3367 = local write "单选_第39路"(w105) -> ()
              n3368 = local write "单选_第40路"(w105) -> ()
              n3369 = local write "单选_第41路"(w105) -> ()
              n3370 = local write "单选_第42路"(w105) -> ()
              n3371 = local write "单选_第43路"(w105) -> ()
              n3372 = local write "单选_第44路"(w105) -> ()
              n3373 = local write "单选_第45路"(w105) -> ()
              n3374 = local write "单选_第46路"(w105) -> ()
              n3375 = local write "单选_第47路"(w105) -> ()
              n3376 = local write "单选_第48路"(w105) -> ()
              n3377 = local write "单选_第49路"(w105) -> ()
              n3378 = local write "单选_第50路"(w105) -> ()
              n3379 = local write "单选_第51路"(w105) -> ()
              n3380 = local write "单选_第52路"(w105) -> ()
              n3381 = local write "单选_第53路"(w105) -> ()
              n3382 = local write "单选_第54路"(w105) -> ()
              n3383 = local write "单选_第55路"(w105) -> ()
              n3384 = local write "单选_第56路"(w105) -> ()
              n3385 = local write "单选_第57路"(w105) -> ()
              n3386 = local write "单选_第58路"(w105) -> ()
              n3387 = local write "单选_第59路"(w105) -> ()
              n3388 = local write "单选_第60路"(w105) -> ()
              n3389 = local write "单选_第61路"(w105) -> ()
              n3390 = local write "单选_第62路"(w105) -> ()
              n3391 = local write "单选_第63路"(w105) -> ()
              n3392 = local write "单选_第64路"(w105) -> ()
              n3393 = local write "单选_第71路"(w105) -> ()
              n3394 = local write "单选_第79路"(w105) -> ()
              n3395 = local write "单选_第65路"(w105) -> ()
              n3396 = local write "单选_第66路"(w105) -> ()
              n3397 = local write "单选_第67路"(w105) -> ()
              n3398 = local write "单选_第68路"(w105) -> ()
              n3399 = local write "单选_第69路"(w105) -> ()
              n3400 = local write "单选_第70路"(w105) -> ()
              n3401 = local write "单选_第72路"(w105) -> ()
              n3402 = local write "单选_第73路"(w105) -> ()
              n3403 = local write "单选_第74路"(w105) -> ()
              n3404 = local write "单选_第75路"(w105) -> ()
              n3405 = local write "单选_第76路"(w105) -> ()
              n3406 = local write "单选_第77路"(w105) -> ()
              n3407 = local write "单选_第78路"(w105) -> ()
              n3408 = local write "单选_第80路"(w105) -> ()
            }
            frame 37 {
              w106 = TRUE
              w107 = FALSE ("单选_第41路")
              n3409 = local write "单选_第1路"(w106) -> ()
              n3410 = local write "单选_第2路"(w106) -> ()
              n3411 = local write "单选_第3路"(w106) -> ()
              n3412 = local write "单选_第4路"(w106) -> ()
              n3413 = local write "单选_第5路"(w106) -> ()
              n3414 = local write "单选_第6路"(w106) -> ()
              n3415 = local write "单选_第7路"(w106) -> ()
              n3416 = local write "单选_第8路"(w106) -> ()
              n3417 = local write "单选_第9路"(w106) -> ()
              n3418 = local write "单选_第10路"(w106) -> ()
              n3419 = local write "单选_第11路"(w106) -> ()
              n3420 = local write "单选_第12路"(w106) -> ()
              n3421 = local write "单选_第13路"(w106) -> ()
              n3422 = local write "单选_第14路"(w106) -> ()
              n3423 = local write "单选_第15路"(w106) -> ()
              n3424 = local write "单选_第16路"(w106) -> ()
              n3425 = local write "单选_第17路"(w106) -> ()
              n3426 = local write "单选_第18路"(w106) -> ()
              n3427 = local write "单选_第19路"(w106) -> ()
              n3428 = local write "单选_第20路"(w106) -> ()
              n3429 = local write "单选_第21路"(w106) -> ()
              n3430 = local write "单选_第22路"(w106) -> ()
              n3431 = local write "单选_第23路"(w106) -> ()
              n3432 = local write "单选_第24路"(w106) -> ()
              n3433 = local write "单选_第25路"(w106) -> ()
              n3434 = local write "单选_第26路"(w106) -> ()
              n3435 = local write "单选_第27路"(w106) -> ()
              n3436 = local write "单选_第28路"(w106) -> ()
              n3437 = local write "单选_第29路"(w106) -> ()
              n3438 = local write "单选_第30路"(w106) -> ()
              n3439 = local write "单选_第31路"(w106) -> ()
              n3440 = local write "单选_第32路"(w106) -> ()
              n3441 = local write "单选_第33路"(w106) -> ()
              n3442 = local write "单选_第34路"(w106) -> ()
              n3443 = local write "单选_第35路"(w106) -> ()
              n3444 = local write "单选_第36路"(w106) -> ()
              n3445 = local write "单选_第37路"(w106) -> ()
              n3446 = local write "单选_第38路"(w107) -> ()
              n3447 = local write "单选_第39路"(w107) -> ()
              n3448 = local write "单选_第40路"(w107) -> ()
              n3449 = local write "单选_第41路"(w107) -> ()
              n3450 = local write "单选_第42路"(w107) -> ()
              n3451 = local write "单选_第43路"(w107) -> ()
              n3452 = local write "单选_第44路"(w107) -> ()
              n3453 = local write "单选_第45路"(w107) -> ()
              n3454 = local write "单选_第46路"(w107) -> ()
              n3455 = local write "单选_第47路"(w107) -> ()
              n3456 = local write "单选_第48路"(w107) -> ()
              n3457 = local write "单选_第49路"(w107) -> ()
              n3458 = local write "单选_第50路"(w107) -> ()
              n3459 = local write "单选_第51路"(w107) -> ()
              n3460 = local write "单选_第52路"(w107) -> ()
              n3461 = local write "单选_第53路"(w107) -> ()
              n3462 = local write "单选_第54路"(w107) -> ()
              n3463 = local write "单选_第55路"(w107) -> ()
              n3464 = local write "单选_第56路"(w107) -> ()
              n3465 = local write "单选_第57路"(w107) -> ()
              n3466 = local write "单选_第58路"(w107) -> ()
              n3467 = local write "单选_第59路"(w107) -> ()
              n3468 = local write "单选_第60路"(w107) -> ()
              n3469 = local write "单选_第61路"(w107) -> ()
              n3470 = local write "单选_第62路"(w107) -> ()
